vi "Baud Rate To Value.vi"(11 "Baud Rate":T1) -> (3 "Baud Rate Value":u32)   [LabVIEW 2013, in "LVH-LINX.lvlib"]
doc: "Convert Baud Rate control to U32 value."
uses:
  <vilib>/LabVIEW Hacker/LINX/LVH-LINX.lvlib
  <vilib>/LabVIEW Hacker/LINX/Private/Type Defs/Baud Rate.ctl
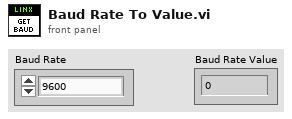
[diagram p1: front panel]
types:
  T1 = typedef "LVH-LINX.lvlib/Baud Rate.ctl" = enum16{"9600", "14400", "19200", "28800", "38400", "57600", "115200"}
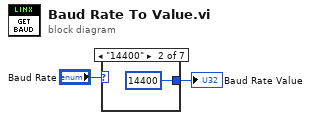
[diagram p0: block diagram]
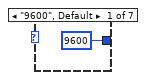
[diagram p2: hidden frame]
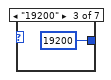
[diagram p3: hidden frame]
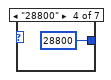
[diagram p4: hidden frame]
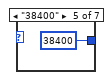
[diagram p5: hidden frame]
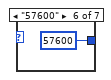
[diagram p6: hidden frame]
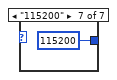
[diagram p7: hidden frame]
diagram:
  n1 = case shown="\"14400\"" "Baud Rate" {
    tunnel: [u32 9600 u32 14400 u32 19200 u32 28800 u32 38400 u32 57600 u32 115200] -> w1
    frame "9600", Default {
    }
    frame "14400" {
    }
    frame "19200" {
    }
    frame "28800" {
    }
    frame "38400" {
    }
    frame "57600" {
    }
    frame "115200" {
    }
  }
  "Baud Rate Value" <- w1
